vi "Initial State Controls Example.vi"() -> ()   [LabVIEW 2018]
uses:
  <vilib>/Initial State by Tektronix/Tektronix, Initial State IoT Streaming SDK/Controls/IS Data Point TypeDef (String).ctl
  <extravilib>/ChannelInstances/Tag-c(bool,i32,str)/Write With Abort.vi
  <extravilib>/ChannelInstances/Tag-c(bool,i32,str)/Read With Abort.vi
  <extravilib>/ChannelInstances/Tag-c(bool,i32,str)/Instantiate.vi
  <extravilib>/ChannelInstances/Tag-c(bool,i32,str)/Endpoint.vi
  <extravilib>/ChannelInstances/Tag-c(bool,i32,str)/EndpointRead.vi
  <extravilib>/ChannelInstances/Tag-c(bool,i32,str).lvlib
panel:
  in  "Access Key":string="<YOUR ACCESS KEY>"
  in  "Bucket Key":string="<YOUR BUCKET KEY>"
  out "Running?":i32
  in  "stop":bool
  in  "Slide":bool
  in  "Rocker Toggle":bool
  in  "Check Box Toggle Switch":bool
  in  "Radio Buttons":enum32{"Item 0", "Item 1"}(radio)
  in  "Button":bool
  in  "Combo Box":string(combo)
  in  "Arbitrary String":string
  in  "Knob":dbl(knob) scale=0.0..10.0
  in  "Vertical Slider Input":dbl(slide) scale=0.0..10.0
  in  "Horizontal Slider Input":dbl(slide) scale=0.0..10.0
  in  "Number Input":dbl
  # "String"
  # "Numeric"
  # "Boolean"
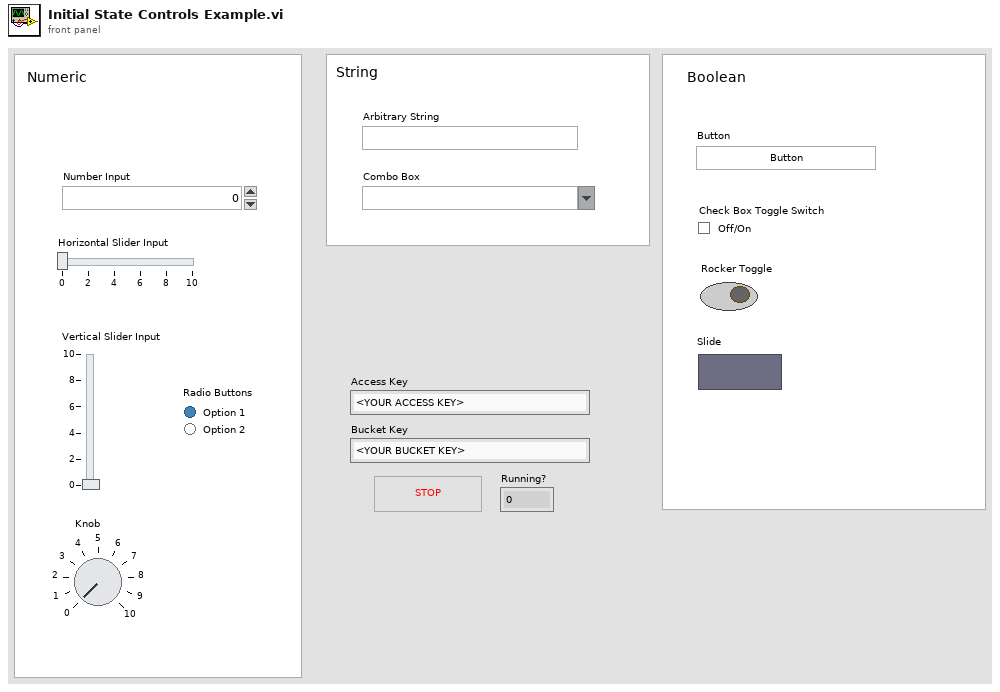
[diagram p1: front panel]
types:
  T1 = typedef "IS Data Point TypeDef (String).ctl" = cluster{"key":string, "value":string, "epoch":dbl}
  T2 = typedef "IS Session.ctl" = cluster{"Access Key":string, "HTTP Client Handle":T3}
  T3 = typedef "LabVIEWHTTPClient.lvlib/ClientHandle.ctl" = refnum<k1>
  T4 = typedef "IS Bucket Session.ctl" = cluster{"Bucket Key":string}
  T5 = typedef "Tag-c(bool,i32,str).lvlib/))Channel.ctl" = refnum<queue>
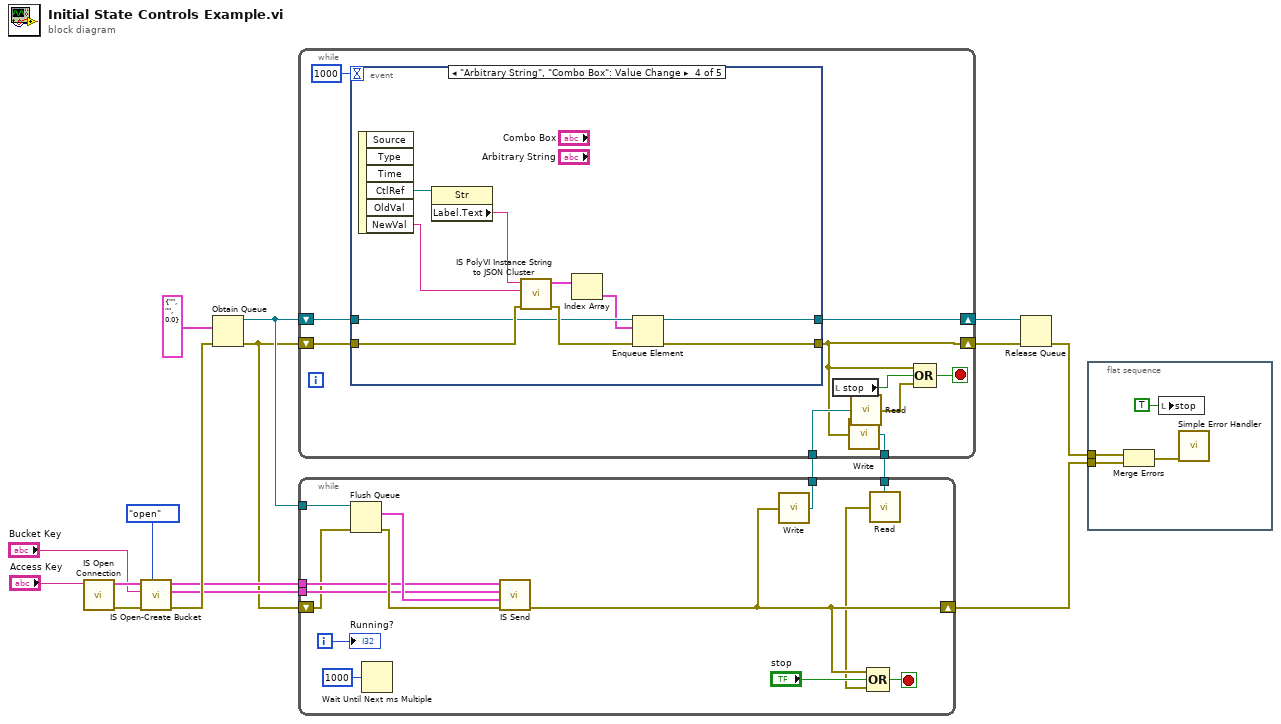
[diagram p0: block diagram]
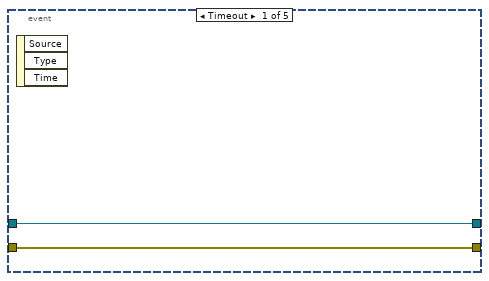
[diagram p2: hidden frame]
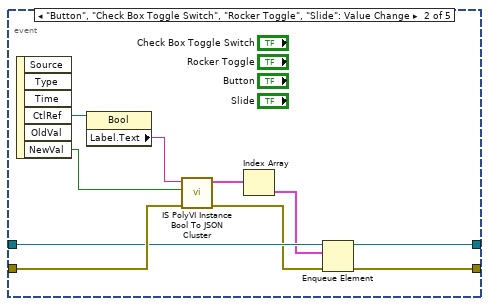
[diagram p3: hidden frame]
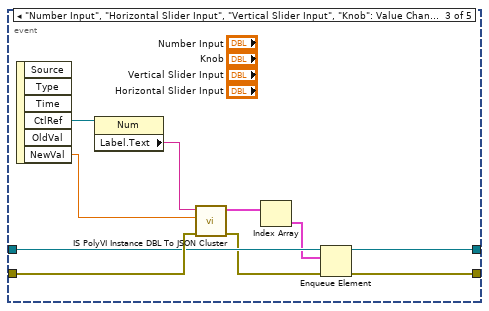
[diagram p4: hidden frame]
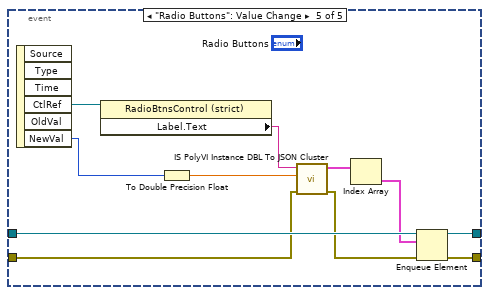
[diagram p5: hidden frame]
diagram:
  n1 = call <vilib>:"IS Open Connection.vi"("Access Key"="Access Key") -> ("error out"=w16:errorcluster, "IS Session"=w15:T2)  [unwired: 9 in]
  n2 = call <vilib>:"IS Open-Create Bucket.vi"("Operation (0: open)"=enum16{"open", "create"}."open", "error in (no error)"=w16, "Bucket Key (Optional)"="Bucket Key", "IS Session In"=w15) -> ("error IO"=w12:errorcluster, "IS Bucket Session"=w9:T4, "IS Session Out"=w10:T2)  [unwired: 5 in]
  n3 = Obtain Queue(element data type=T1 {"key"="", "value"="", "epoch"=0.0} ("element"), error in (no error)=w12) -> (queue out=w11:refnum<queue>, error out=w3:errorcluster)  [unwired: 3 in, 1 out]
  n4 = flat-sequence {
    tunnel: w5 -> [w21]
    tunnel: w7 -> [w20]
    frame #0 {
      n5 = Merge Errors(w21, w20) -> (w19:errorcluster)
      n6 = local write "stop"(TRUE ("stop")) -> ()
      n7 = call <vilib>:"Simple Error Handler.vi"("error in (no error)"=w19) -> ()  [unwired: 4 in, 5 out]
    }
  }
  n8 = while {
    shift-right: [w25] -> w6
    shift-left: w3 -> [w30]
    shift-right: [w28] -> w4
    shift-left: w11 -> [w31]
    tunnel: w2 -> [w27]
    tunnel: [w22] -> w1
    stop <- w26 stop-if-true
    n9 = event shown="[3] \"Arbitrary String\", \"Combo Box\": Value Change" {
      selector: _ -> [_ _ _ _ _]
      dyn-events: _ -> [_ _ _ _ _]
      timeout: 1000 -> [_ _ _ _ _]
      tunnel: w30 -> [w32 w40 w50 w60 w69]
      tunnel: w31 -> [w33 w39 w49 w57 w72]
      tunnel: [w32 w37 w47 w58 w74] -> w25
      tunnel: [w33 w36 w46 w56 w73] -> w28
      event Timeout {
        n10 = event-data() -> ()  [unwired: 1 in, 3 out]
      }
      event "Button", "Check Box Toggle Switch", "Rocker Toggle", "Slide": Value Change {
        n11 = event-data() -> ("CtlRef"=w42:refnum<vi>, "NewVal"=w43:bool)  [unwired: 1 in, 4 out]
        n12 = property class="Bool"(reference=w42) -> ("Label.Text"=w41:string)  [unwired: 1 in, 2 out]
        n13 = call <vilib>:"IS PolyVI Instance Bool To JSON Cluster .vi"("Error In"=w40, "Stream Value"=w43, "Stream Key"=w41) -> ("Error Out"=w38:errorcluster, "JSON Cluster Array out"=w35:T1[])  [unwired: 7 in]
        n14 = Index Array(array=w35) -> (element=w34:T1)  [unwired: 1 in]
        n15 = Enqueue Element(queue=w39, element=w34, error in (no error)=w38) -> (queue out=w36:refnum<queue>, error out=w37:errorcluster)  [unwired: 1 in, 1 out]
      }
      event "Number Input", "Horizontal Slider Input", "Vertical Slider Input", "Knob": Value Change {
        n16 = event-data() -> ("CtlRef"=w52:refnum<vi>, "NewVal"=w53:dbl)  [unwired: 1 in, 4 out]
        n17 = property class="Num"(reference=w52) -> ("Label.Text"=w51:string)  [unwired: 1 in, 2 out]
        n18 = call <vilib>:"IS PolyVI Instance DBL To JSON Cluster .vi"("Error In"=w50, "Stream Value"=w53, "Stream Key"=w51) -> ("Error Out"=w48:errorcluster, "JSON Cluster Array out"=w45:T1[])  [unwired: 7 in]
        n19 = Index Array(array=w45) -> (element=w44:T1)  [unwired: 1 in]
        n20 = Enqueue Element(queue=w49, element=w44, error in (no error)=w48) -> (queue out=w46:refnum<queue>, error out=w47:errorcluster)  [unwired: 1 in, 1 out]
      }
      event "Arbitrary String", "Combo Box": Value Change {
        n21 = event-data() -> ("CtlRef"=w62:refnum<vi>, "NewVal"=w63:string)  [unwired: 1 in, 4 out]
        n22 = property class="Str"(reference=w62) -> ("Label.Text"=w61:string)  [unwired: 1 in, 2 out]
        n23 = call <vilib>:"IS PolyVI Instance String to JSON Cluster.vi"("Error In"=w60, "Stream Value"=w63, "Stream Key"=w61) -> ("Error Out"=w59:errorcluster, "JSON Cluster Array out"=w55:T1[])  [unwired: 7 in]
        n24 = Index Array(array=w55) -> (element=w54:T1)  [unwired: 1 in]
        n25 = Enqueue Element(queue=w57, element=w54, error in (no error)=w59) -> (queue out=w56:refnum<queue>, error out=w58:errorcluster)  [unwired: 1 in, 1 out]
      }
      event "Radio Buttons": Value Change {
        n26 = event-data() -> ("CtlRef"=w71:refnum<vi>, "NewVal"=w65:enum32{"Item 0", "Item 1"})  [unwired: 1 in, 4 out]
        n27 = property class="RadioBtnsControl (strict)"(reference=w71) -> ("Label.Text"=w70:string)  [unwired: 1 in, 2 out]
        n28 = To Double Precision Float(number=w65) -> (double precision float=w64:dbl)
        n29 = call <vilib>:"IS PolyVI Instance DBL To JSON Cluster .vi"("Error In"=w69, "Stream Value"=w64, "Stream Key"=w70) -> ("Error Out"=w68:errorcluster, "JSON Cluster Array out"=w67:T1[])  [unwired: 7 in]
        n30 = Index Array(array=w67) -> (element=w66:T1)  [unwired: 1 in]
        n31 = Enqueue Element(queue=w72, element=w66, error in (no error)=w68) -> (queue out=w73:refnum<queue>, error out=w74:errorcluster)  [unwired: 1 in, 1 out]
      }
    }
    n32 = local read "stop"() -> (w24:bool)
    n33 = call <extravilib>:"Write.vi"("element"=w25) -> ("channel"=w22:T5)  [unwired: 1 out]
    n34 = call <extravilib>:"Read.vi"("channel"=w27) -> ("element"=w23:errorcluster)  [unwired: 1 in, 1 out]
    n35 = Compound Arithmetic op=OR(w25, w24, w23) -> (w26:bool)
  }
  n36 = while {
    tunnel: w11 -> [w88]
    tunnel: w10 -> [w85]
    tunnel: w9 -> [w84]
    shift-right: [w79] -> w7
    shift-left: w3 -> [w81]
    tunnel: [w80] -> w2
    tunnel: w1 -> [w76]
    i -> [w82]
    stop <- w77 stop-if-true
    n37 = Flush Queue(queue=w88, error in (no error)=w81) -> (remaining elements=w86:T1[], error out=w87:errorcluster)  [unwired: 1 out]
    n38 = Wait Until Next ms Multiple(millisecond multiple=u32 1000) -> ()  [unwired: 1 out]
    n39 = call <vilib>:"IS Send.vi"("error in (no error)"=w87, "JSON Custer Array in"=w86, "IS Bucket Session"=w84, "IS Session in"=w85) -> ("Error out"=w79:errorcluster)  [unwired: 2 in, 5 out]
    n40 = call <extravilib>:"Write.vi"("element"=w79) -> ("channel"=w80:T5)  [unwired: 1 out]
    n41 = call <extravilib>:"Read.vi"("channel"=w76) -> ("element"=w75:errorcluster)  [unwired: 1 in, 1 out]
    n42 = Compound Arithmetic op=OR(w79, "stop", w75) -> (w77:bool)
    "Running?" <- w82
  }
  n43 = Release Queue(queue=w4, error in (no error)=w6) -> (error out=w5:errorcluster)  [unwired: 1 in, 2 out]
